vi "Wavefrom_Graph.vi"() -> ()   [LabVIEW 2020]
panel:
  in  "stop":bool
  out "Waveform Chart":dbl(graph)
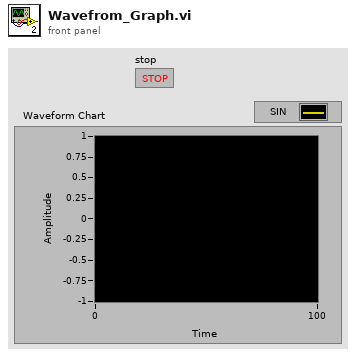
[diagram p1: front panel]
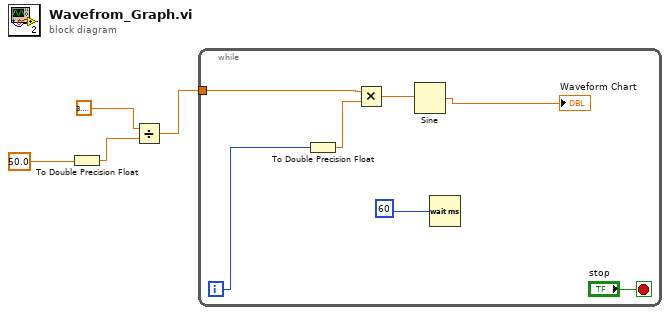
[diagram p0: block diagram]
diagram:
  n1 = To Double Precision Float(number=50.0 ("double precision float")) -> (double precision float=w3:dbl)
  n2 = Divide(x=3.141592653589793, y=w3) -> (x/y=w2:dbl)
  n3 = while {
    tunnel: w2 -> [w11]
    i -> [w10]
    stop <- "stop" stop-if-true
    n4 = To Double Precision Float(number=w10) -> (double precision float=w9:dbl)
    n5 = Multiply(x=w11, y=w9) -> (x*y=w8:dbl)
    n6 = Sine(x=w8) -> (sin(x)=→"Waveform Chart":dbl)
    n7 = Wait (ms)(milliseconds to wait=u32 60 ("millisecond timer value")) -> ()  [unwired: 1 out]
  }
